vi "Is Cooler On.vi"(11 "iCoolerStatus":i32) -> (2 "function return":u32, 3 "iCoolerStatus out":i32)   [LabVIEW 2018, in "AndorSDK.lvlib"]
doc: "EXPNETTYPE unsigned int WINAPI IsCoolerOn(int * iCoolerStatus);"
uses:
  AndorSDK.lvlib
  ATMCD32D.dll
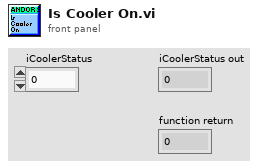
[diagram p1: front panel]
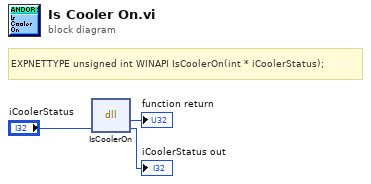
[diagram p0: block diagram]
diagram:
  # "EXPNETTYPE unsigned int WINAPI IsCoolerOn(int * iCoolerStatus);"
  n1 = dll-call lib="PTH2babs E\nPersönliches02 - Arbeit03-HiwijobsLabviewCodelibANDOR\tAndor SDK\nATMCD32D.*" fn="IsCoolerOn"("iCoolerStatus"="iCoolerStatus") -> (→"function return":u32, "iCoolerStatus"=→"iCoolerStatus out":i32)  [unwired: 3 in, 2 out]
